vi "Read Signal Name.vi"(8 "error in (no error)":errorcluster, 11 "NF in":refnum<class "NF.lvclass">) -> (0 "error out":errorcluster, 2 "Signal Name":string, 3 "NF out":refnum<class "NF.lvclass">)   [LabVIEW 2018, in "NF.lvlib" / "NF.lvclass"]
uses:
  NF.lvclass
  NF.lvclass/NF.ctl
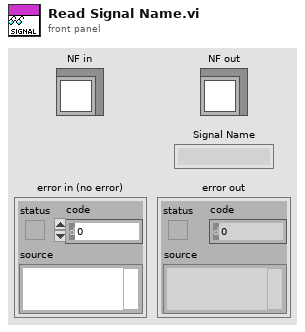
[diagram p1: front panel]
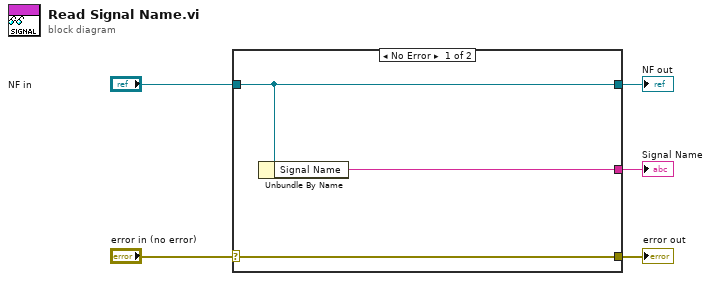
[diagram p0: block diagram]
diagram:
  n1 = case shown="No Error" "error in (no error)" {
    selector: "error in (no error)" -> [w8 w9]
    tunnel: [w8 w9] -> w4
    tunnel: [w7 w10] -> w2
    tunnel: "NF in" -> [w7 w10]
    tunnel: [w6 _] -> w1
    frame No Error {
      n2 = Unbundle By Name(w7) -> ("Signal Name"=w6:string)
    }
    frame Error {
    }
  }
  "error out" <- w4
  "NF out" <- w2
  "Signal Name" <- w1
